vi "Obsługa błędów, LabView 02.10.20.vi"() -> ()   [LabVIEW 2020]
panel:
  out "Final Result":dbl
  out "Random Number":dbl
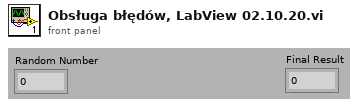
[diagram p1: front panel]
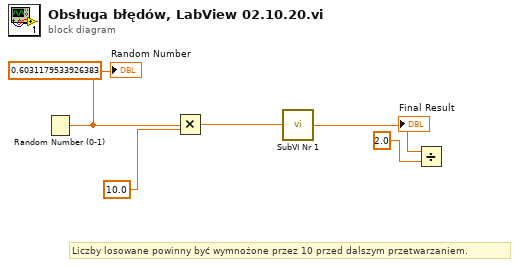
[diagram p0: block diagram]
diagram:
  (unwired) 0.6031179533926383 ("Random Number")
  # "Liczby losowane powinny być wymnożone przez 10 przed dalszym przetwarzaniem."
  n1 = Random Number (0-1)() -> (number: 0 to 1=w3:dbl)
  "Random Number" <- w3
  n2 = Multiply(x=w3, y=10.0) -> (x*y=w1:dbl)
  n3 = call "SubVI Nr 1.vi"("Numeric 2"=w1) -> ("Numeric"=w6:dbl)
  n4 = Divide(x=w6, y=2.0) -> (x/y=→"Final Result":dbl)
